vi "Test Get Project.vi"() -> ()   [LabVIEW 2020]
panel:
  in  "File Path":path
  out "error out":errorcluster
  out "Project Name":string
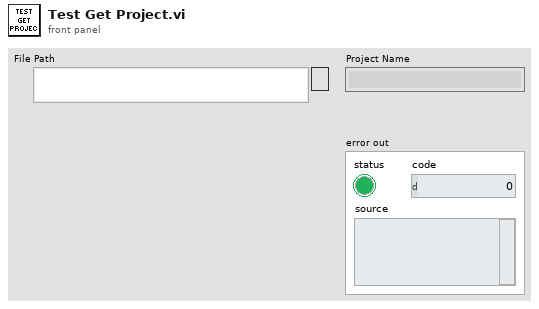
[diagram p1: front panel]
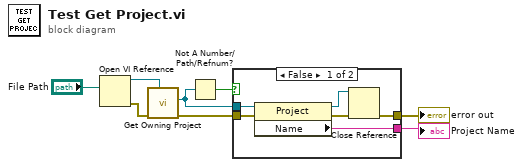
[diagram p0: block diagram]
diagram:
  n1 = Open VI Reference(vi path="File Path") -> (vi reference=w4:refnum<vi>, error out=w7:errorcluster)  [unwired: 5 in]
  n2 = call "Get Owning Project.vi"("VI"=w4, "error in"=w7) -> ("error out"=w8:errorcluster, "Owning Project"=w2:refnum<vi>)  [unwired: 8 in]
  n3 = Not A Number/Path/Refnum?(number/path/refnum=w2) -> (NaN/Path/Refnum?=w1:bool)
  n4 = case shown="False" w1 {
    tunnel: w8 -> [w14 w15]
    tunnel: w2 -> [w11 _]
    tunnel: [w10 _] -> w5
    tunnel: [w12 w15] -> w6
    frame False {
      n5 = property class="Project"(reference=w11, error in=w14) -> (reference out=w9:refnum<vi>, error out=w13:errorcluster, "Name"=w10:string)
      n6 = Close Reference(reference=w9, error in (no error)=w13) -> (error out=w12:errorcluster)
    }
    frame True {
    }
  }
  "Project Name" <- w5
  "error out" <- w6
